vi "Flush Table.vi"(8 "error in":errorcluster) -> (0 "error out":errorcluster)   [LabVIEW 2025, in "CAN-LIN Raw Bus Capture UI.lvlib"]
uses:
  CAN-LIN Raw Bus Capture UI.lvlib
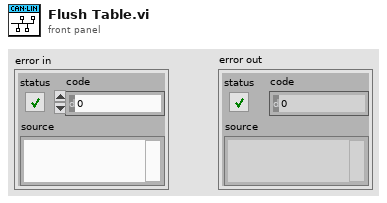
[diagram p1: front panel]
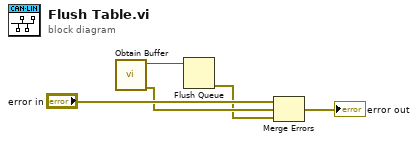
[diagram p0: block diagram]
diagram:
  n1 = call "Obtain Buffer.vi"() -> ("error out"=w2:errorcluster, "Table Queue"=w3:refnum<queue>)  [unwired: 10 in]
  n2 = Flush Queue(queue=w3) -> (error out=w1:errorcluster)  [unwired: 1 in, 2 out]
  n3 = Merge Errors("error in", w2, w1) -> (→"error out":errorcluster)
